vi "01 - Simple Data Network Connection.vi"() -> ()   [LabVIEW 2021]
panel:
  in  "Connect and Send Data":bool
  out "string data":string
  out "data string length":string
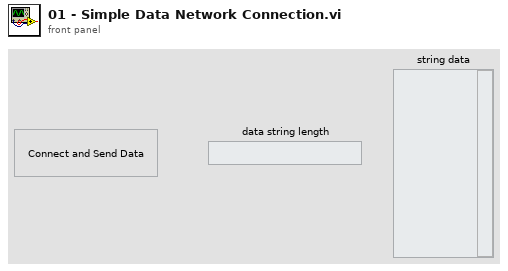
[diagram p1: front panel]
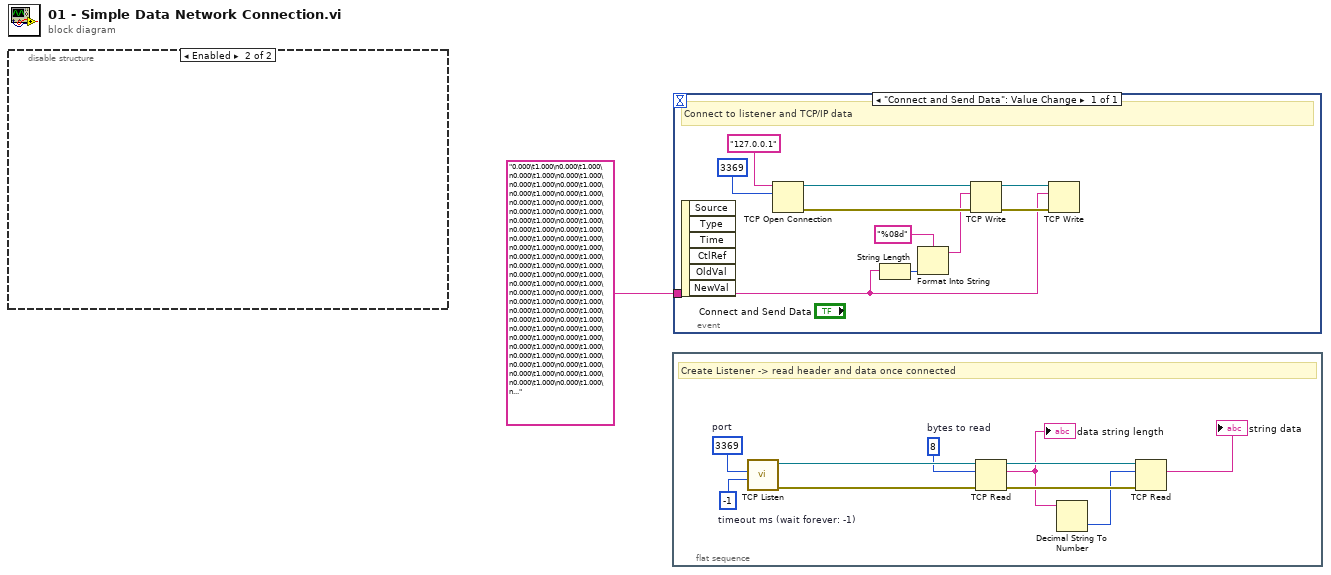
[diagram p0: block diagram]
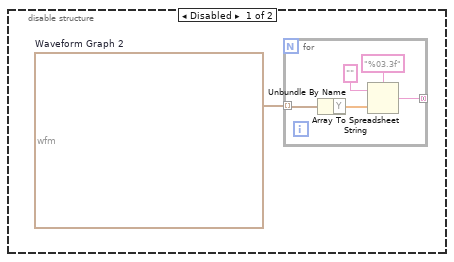
[diagram p2: hidden frame]
diagram:
  n1 = disable-structure shown="Enabled" {
    frame Disabled {
      w2 = waveform(dbl)[] [{"t0"=timestamp(0 s since 1904-01-01), "dt"=0.001, "Y"=array[1000 elements]}, {"t0"=timestamp(0 s since 1904-01-01), "dt"=0.001, "Y"=array[1000 elements]}]  # Waveform Graph 2
      n2 = for {
        tunnel: w2 -> [w7] mode=indexing
        tunnel: [w5] -> _ mode=concatenating
        n3 = Unbundle By Name(w7) -> ("Y"=w6:dbl[])
        n4 = Array To Spreadsheet String(delimiter (Tab)="%03.3f" ("format string"), array=w6, 3:"" ("format string")) -> (spreadsheet string=w5:string)
      }
    }
    frame Enabled {
    }
  }
  n5 = flat-sequence {
    frame #0 {
      w8 = -1  # timeout ms (wait forever: -1)
      w13 = u16 3369  # port
      w14 = 8  # bytes to read
      # "Create Listener -> read header and data once connected"
      n6 = call <vilib>:"TCP Listen.vi"("timeout ms (wait forever: -1)"=w8, "port"=w13) -> ("error out"=w17:errorcluster, "connection ID"=w15:refnum<k5>)  [unwired: 5 in, 3 out]
      n7 = TCP Read(connection ID=w15, bytes to read=w14, error in (no error)=w17) -> (connection ID out=w12:refnum<k5>, data out=w11:string, error out=w16:errorcluster)  [unwired: 2 in]
      "data string length" <- w11
      n8 = Decimal String To Number(string=w11) -> (number=w10:i32)  [unwired: 2 in, 1 out]
      n9 = TCP Read(connection ID=w12, bytes to read=w10, error in (no error)=w16) -> (data out=→"string data":string)  [unwired: 2 in, 2 out]
    }
  }
  n10 = event shown="[0] \"Connect and Send Data\": Value Change" {
    selector: _ -> [_]
    dyn-events: _ -> [_]
    timeout: _ -> [_]
    tunnel: "0.000\t1.000\n0.000\t1.000\n0.000\t1.000\n0.000\t1.000\n0.000\t1.000\n0.000\t1.000\n0.000\t1.000\n0.000\t1.000\n0.000\t1.000\n0.000\t1.000\n0.000\t1.000\n0.000\t1.000\n0.000\t1.000\n0.000\t1.000\n0.000\t1.000\n0.000\t1.000\n0.000\t1.000\n0.000\t1.000\n0.000\t1.000\n0.000\t1.000\n0.000\t1.000\n0.000\t1.000\n0.000\t1.000\n0.000\t1.000\n0.000\t1.000\n0.000\t1.000\n0.000\t1.000\n0.000\t1.000\n0.000\t1.000\n0.000\t1.000\n0.000\t1.000\n0.000\t1.000\n0.000\t1.000\n0.000\t1.000\n0.000\t1.000\n0.000\t1.000\n0.000\t1.000\n0.000\t1.000\n0.000\t1.000\n0.000\t1.000\n0.000\t1.000\n0.000\t1.000\n0.000\t1.000\n0.000\t1.000\n0.000\t1.000\n0.000\t1.000\n0.000\t1.000\n0.000\t1.000\n0.000\t1.000\n0.000\t1.000\n0.000\t1.000\n0.000\t1.000\n0.000\t1.000\n0.000\t1.000\n0.000\t1.000\n0.000\t1.000\n0.000\t1.000\n0.000\t1.000\n0.500\t1.000\n1.000\t1.000\n0.500\t1.000\n0.000\t1.000\n0.000\t1.000\n0.000\t1.000\n0.000\t1.000\n0.000\t1.000\n0.000\t1.000\n0.000\t1.000\n0.000\t1.000\n0.000\t1.000\n0.000\t1.000\n0.000\t1.000\n0.000\t1.000\n0.000\t1.000\n0.000\t1.000\n0.000\t1.000\n0.000\t1.000\n0.000\t1.000\n0.000\t1.000\n0.000\t1.000\n0.000\t1.000\n0.000\t1.000\n0.000\t1.000\n0.000\t1.000\n0.000\t1.000\n0.000\t1.000\n0.000\t1.000\n0.000\t1.000\n0.000\t1.000\n0.000\t1.000\n0.000\t1.000\n0.000\t1.000\n0.000\t1.000\n0.000\t1.000\n0.000\t1.000\n0.000\t1.000\n0.000\t1.000\n0.000\t1.000\n0.000\t1.000\n0.000\t1.000\n0.000\t1.000\n0.000\t1.000\n0.000\t1.000\n0.000\t1.000\n0.000\t1.000\n0.000\t1.000\n0.000\t1.000\n0.000\t1.000\n0.000\t1.000\n0.000\t1.000\n0.000\t1.000\n0.000\t1.000\n0.000\t1.000\n0.000\t1.000\n0.000\t1.000\n0.000\t1.000\n0.000\t1.000\n0.000\t1.000\n0.000\t1.000\n0.000\t1.000\n0.000\t1.000\n0.000\t1.000\n0.000\t1.000\n0.000\t1.000\n0.000\t1.000\n0.000\t1.000\n0.000\t1.000\n0.000\t1.000\n0.000\t1.000\n0.000\t1.000\n0.000\t1.000\n0.000\t1.000\n0.000\t1.000\n0.000\t1.000\n0.000\t1.000\n0.000\t1.000\n0.000\t1.000\n0.000\t1.000\n0.000\t1.000\n0.000\t1.000\n0.000\t1.000\n0.000\t1.000\n0.000\t1.000\n0.000\t1.000\n0.000\t1.000\n0.000\t1.000\n0.000\t1.000\n0.000\t1.000\n0.000\t1.000\n0.000\t1.000\n0.000\t1.000\n0.000\t1.000\n0.000\t1.000\n0.000\t1.000\n0.000\t1.000\n0.000\t1.000\n0.000\t1.000\n0.000\t1.000\n0.000\t1.000\n0.000\t1.000\n0.000\t1.000\n0.000\t1.000\n0.000\t1.000\n0.000\t1.000\n0.000\t1.000\n0.000\t1.000\n0.000\t1.000\n0.000\t1.000\n0.000\t1.000\n0.000\t1.000\n0.000\t1.000\n0.000\t1.000\n0.000\t1.000\n0.000\t1.000\n0.000\t1.000\n0.000\t1.000\n0.000\t1.000\n0.000\t1.000\n0.000\t1.000\n0.000\t1.000\n0.000\t1.000\n0.000\t1.000\n0.000\t1.000\n0.000\t1.000\n0.000\t1.000\n0.000\t1.000\n0.000\t1.000\n0.000\t1.000\n0.000\t1.000\n0.000\t1.000\n0.000\t1.000\n0.000\t1.000\n0.000\t1.000\n0.000\t1.000\n0.000\t1.000\n0.000\t1.000\n0.000\t1.000\n0.000\t0.999\n0.000\t0.999\n0.000\t0.999\n0.000\t0.999\n0.000\t0.999\n0.000\t0.999\n0.000\t0.998\n0.000\t0.998\n0.000\t0.998\n0.000\t0.997\n0.000\t0.997\n0.000\t0.996\n0.000\t0.996\n0.000\t0.995\n0.000\t0.994\n0.000\t0.993\n0.000\t0.992\n0.000\t0.991\n0.000\t0.990\n0.000\t0.989\n0.000\t0.987\n0.000\t0.986\n0.000\t0.984\n0.000\t0.982\n0.000\t0.980\n0.000\t0.977\n0.000\t0.974\n0.000\t0.972\n0.000\t0.968\n0.000\t0.965\n0.000\t0.961\n0.000\t0.957\n0.000\t0.953\n0.000\t0.948\n0.000\t0.943\n0.000\t0.937\n0.000\t0.932\n0.000\t0.925\n0.000\t0.919\n0.000\t0.912\n0.000\t0.904\n0.000\t0.896\n0.000\t0.888\n0.000\t0.879\n0.000\t0.870\n0.000\t0.860\n0.000\t0.850\n0.000\t0.840\n0.000\t0.829\n0.000\t0.817\n0.000\t0.805\n0.000\t0.793\n0.000\t0.780\n0.000\t0.766\n0.000\t0.753\n0.000\t0.739\n0.000\t0.724\n0.000\t0.709\n0.000\t0.694\n0.000\t0.678\n0.000\t0.662\n0.000\t0.646\n0.000\t0.630\n0.000\t0.613\n0.000\t0.596\n0.000\t0.579\n0.000\t0.562\n0.000\t0.545\n0.000\t0.527\n0.000\t0.510\n0.000\t0.493\n0.000\t0.475\n0.000\t0.458\n0.000\t0.440\n0.000\t0.423\n0.000\t0.406\n0.000\t0.389\n0.000\t0.373\n0.000\t0.356\n0.000\t0.340\n0.000\t0.324\n0.000\t0.308\n0.000\t0.293\n0.000\t0.278\n0.000\t0.263\n0.000\t0.249\n0.000\t0.235\n0.000\t0.222\n0.000\t0.209\n0.000\t0.197\n0.000\t0.185\n0.000\t0.173\n0.000\t0.162\n0.000\t0.151\n0.000\t0.141\n0.000\t0.131\n0.000\t0.122\n0.000\t0.113\n0.000\t0.104\n0.000\t0.096\n0.000\t0.089\n0.000\t0.082\n0.000\t0.075\n0.000\t0.069\n0.000\t0.063\n0.000\t0.058\n0.000\t0.052\n0.000\t0.048\n0.000\t0.043\n0.000\t0.039\n0.000\t0.035\n0.000\t0.032\n0.000\t0.029\n0.000\t0.026\n0.000\t0.023\n0.000\t0.020\n0.000\t0.018\n0.000\t0.016\n0.000\t0.014\n0.000\t0.013\n0.000\t0.011\n0.000\t0.010\n0.000\t0.009\n0.000\t0.007\n0.000\t0.007\n0.000\t0.006\n0.000\t0.005\n0.000\t0.004\n0.000\t0.004\n0.000\t0.003\n0.000\t0.003\n0.000\t0.002\n0.000\t0.002\n0.000\t0.002\n0.000\t0.001\n0.000\t0.001\n0.000\t0.001\n0.000\t0.001\n0.000\t0.001\n0.000\t0.001\n0.000\t0.000\n0.000\t0.000\n0.000\t0.000\n0.000\t0.000\n0.000\t0.000\n0.000\t0.000\n0.000\t0.000\n0.000\t0.000\n0.000\t0.000\n0.000\t0.000\n0.000\t0.000\n0.000\t0.000\n0.000\t0.000\n0.000\t0.000\n0.000\t0.000\n0.000\t0.000\n0.000\t0.000\n0.000\t0.000\n0.000\t0.000\n0.000\t0.000\n0.000\t0.000\n0.000\t0.000\n0.000\t0.000\n0.000\t0.000\n0.000\t0.000\n0.000\t0.000\n0.000\t0.000\n0.000\t0.000\n0.000\t0.000\n0.000\t0.000\n0.000\t0.000\n0.000\t0.000\n0.000\t0.000\n0.000\t0.000\n0.000\t0.000\n0.000\t0.000\n0.000\t0.000\n0.000\t0.000\n0.000\t0.000\n0.000\t0.000\n0.000\t0.000\n0.000\t0.000\n0.000\t0.000\n0.000\t0.000\n0.000\t0.000\n0.000\t0.000\n0.000\t0.000\n0.000\t0.000\n0.000\t0.000\n0.000\t0.000\n0.000\t0.000\n0.000\t0.000\n0.000\t0.000\n0.000\t0.000\n0.000\t0.000\n0.000\t0.000\n0.000\t0.000\n0.000\t0.000\n0.000\t0.000\n0.000\t0.000\n0.000\t0.000\n0.000\t0.000\n0.000\t0.000\n0.000\t0.000\n0.000\t0.000\n0.000\t0.000\n0.000\t0.000\n0.000\t0.000\n0.000\t0.000\n0.000\t0.000\n0.000\t0.000\n0.000\t0.000\n0.000\t0.000\n0.000\t0.000\n0.000\t0.000\n0.000\t0.000\n0.000\t0.000\n0.000\t0.000\n0.000\t0.000\n0.000\t0.000\n0.000\t0.000\n0.000\t0.000\n0.000\t0.000\n0.000\t0.000\n0.000\t0.000\n0.000\t0.000\n0.000\t0.000\n0.000\t0.000\n0.000\t0.000\n0.000\t0.000\n0.000\t0.000\n0.000\t0.000\n0.000\t0.000\n0.000\t0.000\n0.000\t0.000\n0.000\t0.000\n0.000\t0.000\n0.000\t0.000\n0.000\t0.000\n0.000\t0.000\n0.000\t0.000\n0.000\t0.000\n0.000\t0.000\n0.000\t0.000\n0.000\t0.000\n0.000\t0.000\n0.000\t0.000\n0.000\t0.000\n0.000\t0.000\n0.000\t0.000\n0.000\t0.000\n0.000\t0.000\n0.000\t0.000\n0.000\t0.000\n0.000\t0.000\n0.000\t0.000\n0.000\t0.000\n0.000\t0.000\n0.000\t0.000\n0.000\t0.000\n0.000\t0.000\n0.000\t0.000\n0.000\t0.000\n0.000\t0.000\n0.000\t0.000\n0.000\t0.000\n0.000\t0.000\n0.000\t0.000\n0.000\t0.000\n0.000\t0.000\n0.000\t0.000\n0.000\t0.000\n0.000\t0.000\n0.000\t0.000\n0.000\t0.000\n0.000\t0.000\n0.000\t0.000\n0.000\t0.000\n0.000\t0.000\n0.000\t0.000\n0.000\t0.000\n0.000\t0.000\n0.000\t0.000\n0.000\t0.000\n0.000\t0.000\n0.000\t0.000\n0.000\t0.000\n0.000\t0.000\n0.000\t0.000\n0.000\t0.000\n0.000\t0.000\n0.000\t0.000\n0.000\t0.000\n0.000\t0.000\n0.000\t0.000\n0.000\t0.000\n0.000\t0.000\n0.000\t0.000\n0.000\t0.000\n0.000\t0.000\n0.000\t0.000\n0.000\t0.000\n0.000\t0.000\n0.000\t0.000\n0.000\t0.000\n0.000\t0.000\n0.000\t0.000\n0.000\t0.000\n0.000\t0.000\n0.000\t0.000\n0.000\t0.000\n0.000\t0.000\n0.000\t0.000\n0.000\t0.000\n0.000\t0.000\n0.000\t0.000\n" ("address") -> [w21]
    event "Connect and Send Data": Value Change {
      # "Connect to listener and TCP/IP data"
      n11 = event-data() -> ()  [unwired: 1 in, 6 out]
      n12 = TCP Open Connection(address="127.0.0.1", remote port or service name=u16 3369) -> (connection ID=w23:refnum<k5>, error out=w27:errorcluster)  [unwired: 3 in]
      n13 = String Length(string=w21) -> (length=w20:i32)
      n14 = Format Into String(format string="%08d", w20) -> (resulting string=w19:string)  [unwired: 2 in, 1 out]
      n15 = TCP Write(connection ID=w23, data in=w19, error in (no error)=w27) -> (connection ID out=w22:refnum<k5>, error out=w26:errorcluster)  [unwired: 1 in, 1 out]
      n16 = TCP Write(connection ID=w22, data in=w21, error in (no error)=w26) -> ()  [unwired: 1 in, 3 out]
    }
  }
